vi "RT-FPGA9205.vi"(5 "9205采样率":u32=32000, 9 "9205采样点数":u32=32000, 11 "错误输入":errorcluster) -> (1 "9205电压波形":waveform(sgl)[](array[waveform]), 2 "9205电流波形":waveform(sgl)[](array[waveform]), 4 "FPGA VI引用输出":refnum<k20>, 6 "9205数据":sgl[](array[numeric]), 8 "9205时间t0":timestamp, 10 "9205dt":dbl, 12 "9205fifo flower":bool, 13 "9205fifo over":bool, 14 "9205剩余元素":u32, 15 "错误输出":errorcluster)   [LabVIEW 2013]
uses:
  <vilib>/rvi/interface/common/niFpgaWaitOnOcc.vi
  <vilib>/Utility/error.llb/Error Cluster From Error Code.vi
  <vilib>/rvi/errors/niLvFpgaAdjustHostInterfaceError.vi
  <vilib>/rvi/interface/nirviMethod/nirviMethod.xnode
  <vilib>/rvi/interface/nirviReadWriteControl/nirviReadWriteControl.xnode
  <vilib>/FPGAPlugInAG/Dynamic/niLvFpga_ReadFifo_Dynamic.vi
  <vilib>/rvi/errors/niLvFpgaMergeErrorWithErrorCode.vi
  NiFpgaLv.dll
  <vilib>/rvi/interface/Simulation/niFpgaSimulationCallBeginRW.vi
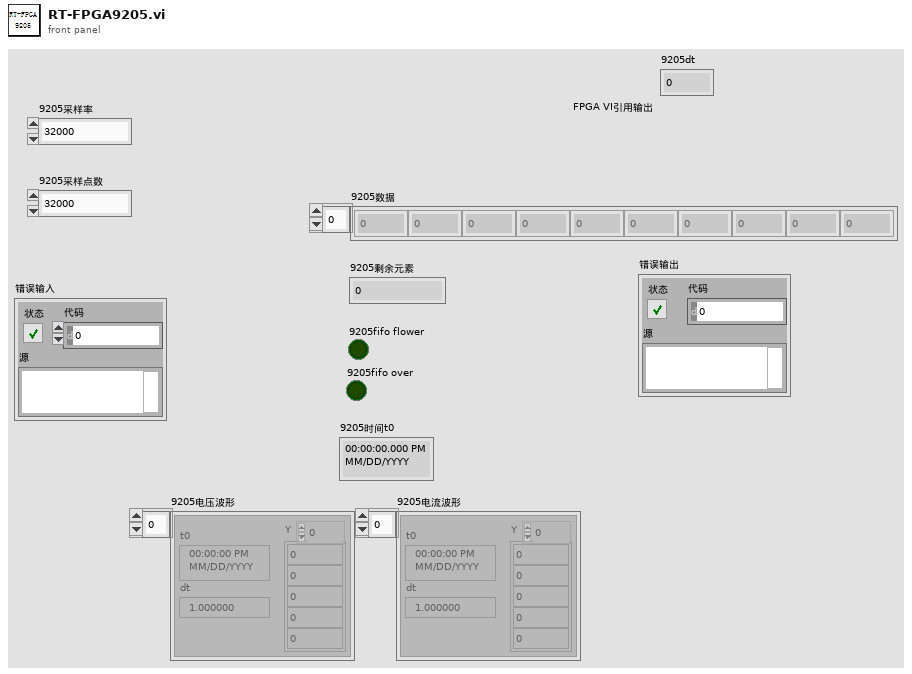
[diagram p1: front panel]
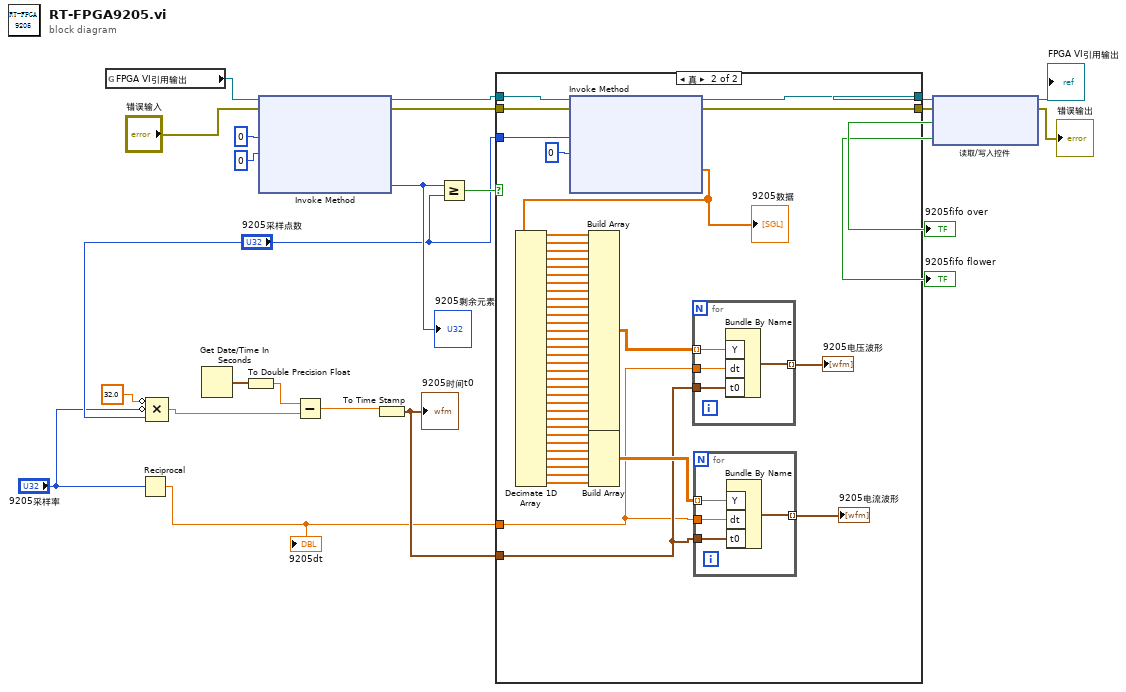
[diagram p0: block diagram]
diagram:
  n1 = global read "RT-FPGA引用全局.vi" "FPGA VI引用输出"() -> (w2:refnum<k20>)
  n2 = Reciprocal(x="9205采样率") -> (1/x=w3:dbl)
  "9205dt" <- w3
  n3 = Compound Arithmetic op=MULTIPLY(invert 32.0 ("值"), invert "9205采样率", "9205采样点数") -> (w7:dbl)
  n4 = Get Date/Time In Seconds() -> (seconds since 1Jan1904=w9:timestamp)
  n5 = To Double Precision Float(number=w9) -> (double precision float=w8:dbl)
  n6 = xnode "Invoke Method"("FPGA VI引用输入"=w2, "错误输入"="错误输入", "元素数量"=u32 0, "超时(ms)"=0) -> ("FPGA VI引用输出"=w20:refnum<k20>, "错误输出"=w16:errorcluster, "剩余元素"=w21:u32)  [unwired: 1 out]
  "9205剩余元素" <- w21
  n7 = Subtract(x=w8, y=w7) -> (x-y=w6:dbl)
  n8 = To Time Stamp(1:w6) -> (0:w5:timestamp)
  "9205时间t0" <- w5
  n9 = Greater Or Equal?(x=w21, y="9205采样点数") -> (x >= y?=w19:bool)
  n10 = case shown="真" w19 {
    tunnel: w20 -> [w25 w70]
    tunnel: "9205采样点数" -> [_ w68]
    tunnel: [w25 w67] -> w18
    tunnel: [w24 w66] -> w17
    tunnel: w16 -> [w24 w65]
    tunnel: w5 -> [_ w28]
    tunnel: w3 -> [_ w27]
    frame False {
    }
    frame True {
      n11 = xnode "Invoke Method"("FPGA VI引用输入"=w70, "错误输入"=w65, "元素数量"=w68, "超时(ms)"=0) -> ("FPGA VI引用输出"=w67:refnum<k20>, "错误输出"=w66:errorcluster, "数据"=w32:sgl[])  [unwired: 1 out]
      "9205数据" <- w32
      n12 = Decimate 1D Array(w32) -> (w64:sgl[], w63:sgl[], w62:sgl[], w61:sgl[], w60:sgl[], w59:sgl[], w58:sgl[], w57:sgl[], w56:sgl[], w55:sgl[], w54:sgl[], w53:sgl[], w52:sgl[], w51:sgl[], w50:sgl[], w49:sgl[], w48:sgl[], w47:sgl[], w46:sgl[], w45:sgl[], w44:sgl[], w43:sgl[], w42:sgl[], w41:sgl[], w40:sgl[], w39:sgl[], w38:sgl[], w37:sgl[], w36:sgl[], w35:sgl[], w34:sgl[], w33:sgl[])
      n13 = Build Array(w64, w63, w62, w61, w60, w59, w58, w57, w56, w55, w54, w53, w52, w51, w50, w49, w48, w47, w46, w45, w44, w43, w42, w41, w40) -> (w31:sgl[][])
      n14 = Build Array(w39, w38, w37, w36, w35, w34, w33) -> (w29:sgl[][])
      n15 = for {
        tunnel: w28 -> [w78]
        tunnel: w27 -> [w77]
        tunnel: w31 -> [w76] mode=indexing
        tunnel: [w75] -> w30 mode=indexing
        n16 = Bundle By Name("Y"=w76, "dt"=w77, "t0"=w78) -> (w75:waveform(sgl))  [unwired: 1 in]
      }
      "9205电压波形" <- w30
      n17 = for {
        tunnel: w28 -> [w74]
        tunnel: w27 -> [w73]
        tunnel: w29 -> [w72] mode=indexing
        tunnel: [w71] -> w26 mode=indexing
        n18 = Bundle By Name("Y"=w72, "dt"=w73, "t0"=w74) -> (w71:waveform(sgl))  [unwired: 1 in]
      }
      "9205电流波形" <- w26
    }
  }
  n19 = xnode "读取/写入控件"("FPGA VI引用输入"=w18, "错误输入"=w17) -> ("FPGA VI引用输出"=→"FPGA VI引用输出":refnum<k20>, "错误输出"=→"错误输出":errorcluster, "9205fifo over"=→"9205fifo over":bool, "9205fifo flower"=→"9205fifo flower":bool)
